vi "_Add Module By Path.vi"(8 "error in":errorcluster, 10 "New Module Name":string, 11 "New Module Folder":path) -> (0 "error out":errorcluster)   [LabVIEW 2020, in "Panther Dasboard Scripting Hooks.lvlib"]
uses:
  Panther Dasboard Scripting Hooks.lvlib
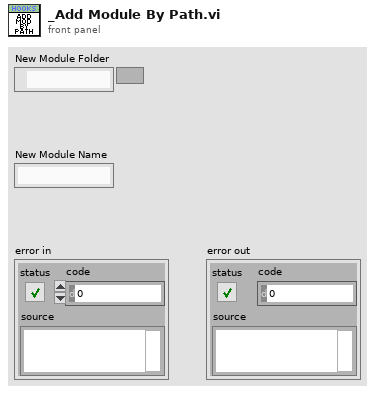
[diagram p1: front panel]
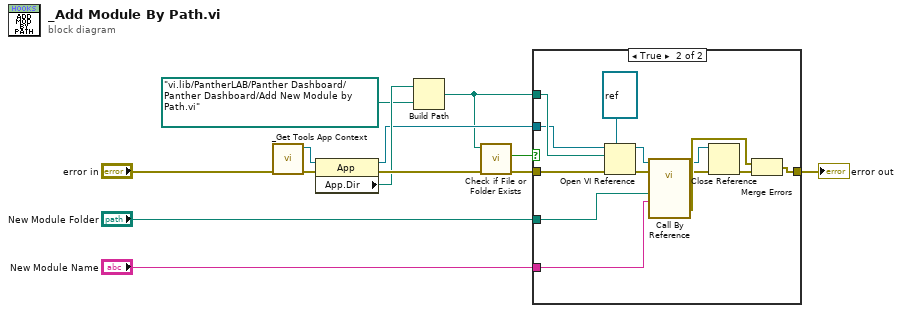
[diagram p0: block diagram]
diagram:
  n1 = call "_Get Tools App Context.vi"("error in"="error in") -> ("error out"=w11:errorcluster, "Application Context"=w4:refnum<vi>)  [unwired: 9 in]
  n2 = property class="App"(reference=w4, error in=w11) -> (reference out=w3:refnum<vi>, error out=w12:errorcluster, "App.Dir"=w6:path)
  n3 = Build Path(base path=w6, name or relative path=path "vi.lib/PantherLAB/Panther Dashboard/Panther Dashboard/Add New Module by Path.vi") -> (appended path=w2:path)
  n4 = call <vilib>:"Check if File or Folder Exists.vi"("error in (no error)"=w12, "path"=w2) -> ("error out"=w9:errorcluster, "file or folder exists?"=w1:bool)  [unwired: 7 in, 1 out]
  n5 = case shown="True" w1 {
    tunnel: [w14 w26] -> w13
    tunnel: w9 -> [w14 w24]
    tunnel: "New Module Name" -> [_ w21]
    tunnel: "New Module Folder" -> [_ w20]
    tunnel: w2 -> [_ w18]
    tunnel: w3 -> [_ w15]
    frame False {
    }
    frame True {
      n6 = Open VI Reference(type specifier VI Refnum (for type only)=refnum<vi> refnum, application reference (local)=w15, vi path=w18, error in (no error)=w24) -> (vi reference=w17:refnum<vi>, error out=w23:errorcluster)  [unwired: 2 in]
      n7 = call-by-ref "?"(reference=w17, error in=w23, "Module Name"=w21, "Module Folder"=w20) -> (reference out=w16:refnum<vi>, error out=w22:errorcluster, 0:"error out"=w27:errorcluster)  [unwired: 9 in]
      n8 = Close Reference(reference=w16, error in (no error)=w22) -> (error out=w25:errorcluster)
      n9 = Merge Errors(w27, w25) -> (w26:errorcluster)
    }
  }
  "error out" <- w13
